vi "working-HostControl_Main.vi"() -> ()   [LabVIEW 2013]
uses:
  Messages.ctl
  PolarCoordTdef.ctl
  GainsTDef.ctl
  Support VIs/setpointCluster.ctl
  <vilib>/MakerHub/KinectOne/Private/Initialize Image [Color].vi
  <vilib>/MakerHub/PS4-Controller/Public/Open First Controller.vi
  Support VIs/bodyGlobal.vi
  <vilib>/MakerHub/KinectOne/KinectOne.lvlib
  <vilib>/MakerHub/PS4-Controller/LMH-PS4.lvlib
panel:
  in  "Reference Colour":u32(colorbox)
  in  "Argument Setpoint":dbl
  in  "Modulus Setpoint":dbl=1.8
  out "Tracked?":bool
  out "index":i32
  in  "Detect Mode":u16(ring) items=["Desperate", "ColourMatch"]
  in  "Cancel Button":bool
  out "Image":T1(plugin-control)
  in  "Kd-Argument":dbl
  in  "Kc-Argument":dbl
  in  "Kd-Modulus":dbl
  in  "Kc-Modulus":dbl
  out "Mod":dbl
  out "Arg":dbl
  in  "IT'S TIME TO":bool
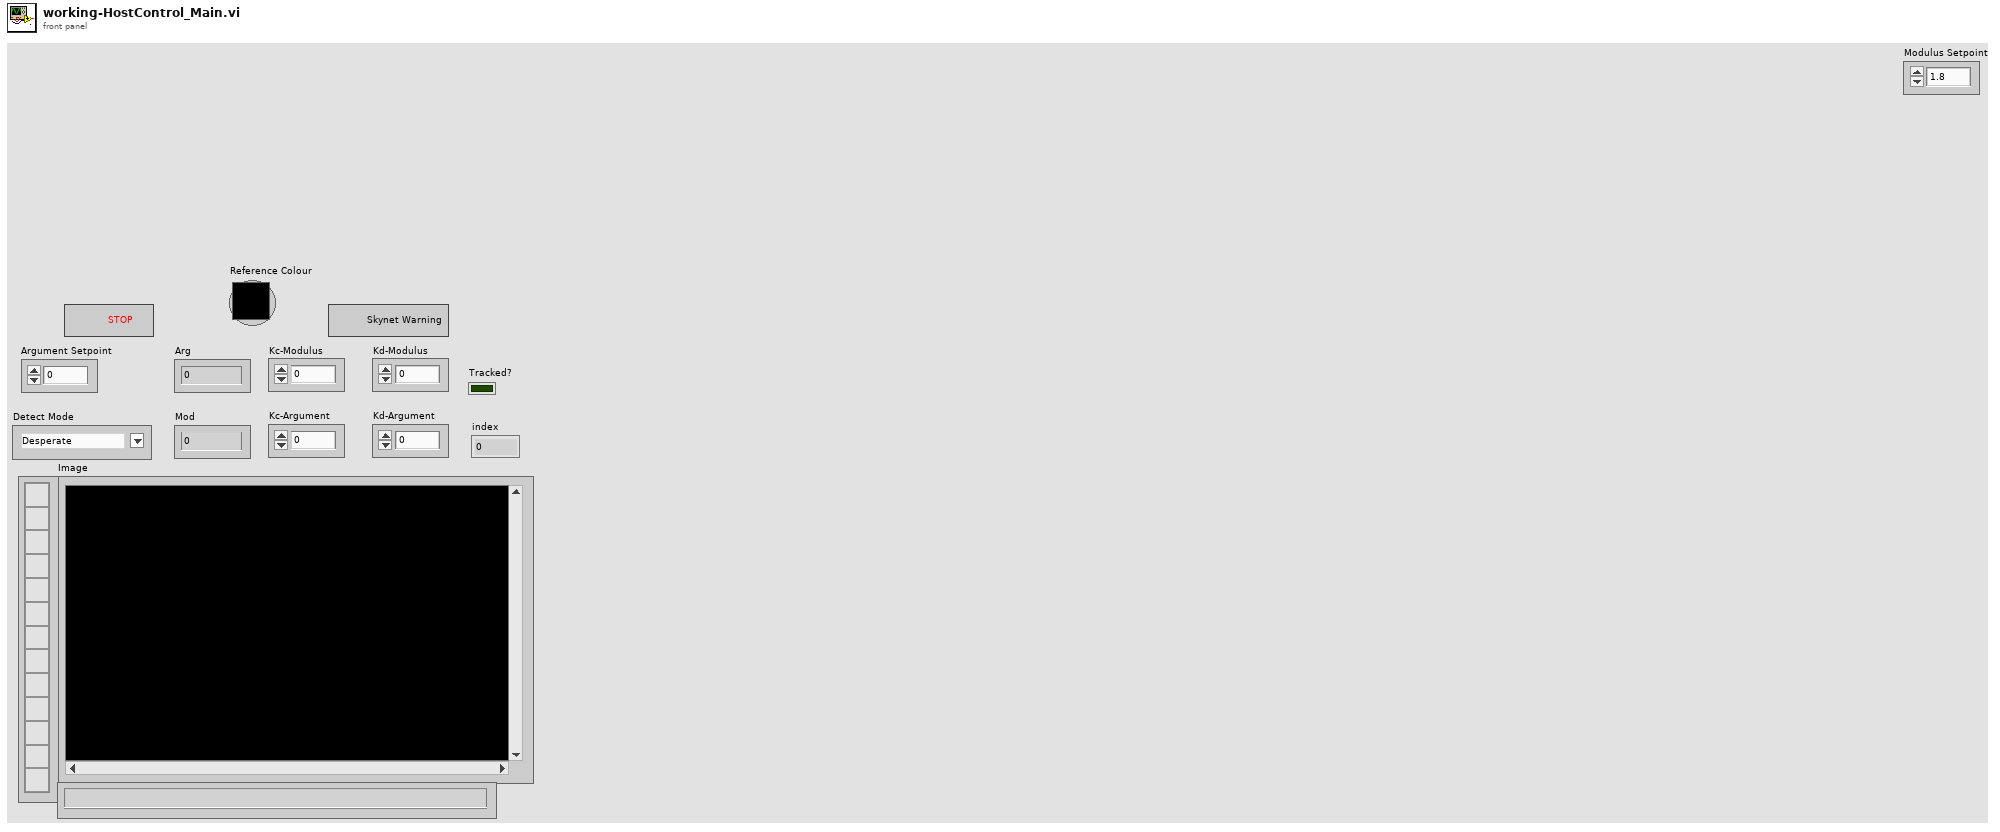
[diagram p1: front panel]
types:
  T1 = typedef "IMAQ Image.ctl" = refnum<image>
  T2 = typedef "Messages.ctl" = cluster{"message data":variant, "message type":enum16{"Stop", "PolarCoordinates", "Gains", "Setpoints"}}
  T3 = typedef "KinectOne.lvlib/KinectSensor References.ctl" = cluster{"KinectSensor":refnum<k24>, "MultiSourceFrameReader":refnum<k24>, "BodyFrameDataInterface":refnum<k24>}
  T4 = typedef "LMH-PS4.lvlib/PS4 Controller Ref.ctl" = cluster{"Controller Ref":refnum<k1>, "PS4 Events Ref":refnum<event-registration>, "Worker Ref":refnum<vi>}
  T5 = enum16{"Stop", "PolarCoordinates", "Gains", "Setpoints"}
  T6 = typedef "PolarCoordTdef.ctl" = cluster{"Argument":dbl, "Modulus":dbl, "trackedState":bool}
  T7 = typedef "KinectOne.lvlib/Joint Position.ctl" = cluster{"Camera Space":cluster{"X":dbl, "Y":dbl, "Z":dbl}, "Color Space":cluster{"X":dbl, "Y":dbl}, "Depth Space":cluster{"X":dbl, "Y":dbl}, "Tracking State":enum16{"NotTracked", "Inferred", "Tracked"}}
  T8 = typedef "setpointCluster.ctl" = cluster{"Modulus Setpoint":dbl, "Argument Setpoint":dbl}
  T9 = typedef "KinectOne.lvlib/BodyData.ctl" = cluster{"ClippedEdges":T10, "HandLeftConfidence":T11, "HandLeftState":T12, "HandRightConfidence":T13, "HandRightState":T14, "IsRestricted":bool, "IsTracked":bool, "JointOrientations":refnum<k24>, "Joints":refnum<k24>, "Lean":refnum<k24>, "LeanTrackingState":T15, "TrackingId":u64}
  T10 = typedef "KinectOne.lvlib/ClippedEdges.ctl" = enum16{"None", "Right", "Left", "Top", "Bottom"}
  T11 = typedef "KinectOne.lvlib/HandLeftConfidence.ctl" = enum16{"Low", "High"}
  T12 = typedef "KinectOne.lvlib/HandLeftState.ctl" = enum16{"Unknown", "NotTracked", "Open", "Closed", "Lasso"}
  T13 = typedef "KinectOne.lvlib/HandRightConfidence.ctl" = enum16{"Low", "High"}
  T14 = typedef "KinectOne.lvlib/HandRightState.ctl" = enum16{"Unknown", "NotTracked", "Open", "Closed", "Lasso"}
  T15 = typedef "KinectOne.lvlib/LeanTrackingState.ctl" = enum16{"NotTracked", "Inferred", "Tracked"}
  T16 = typedef "GainsTDef.ctl" = cluster{"Kc-Modulus":dbl, "Kd-Modulus":dbl, "Kc-Argument":dbl, "Kd-Argument":dbl}
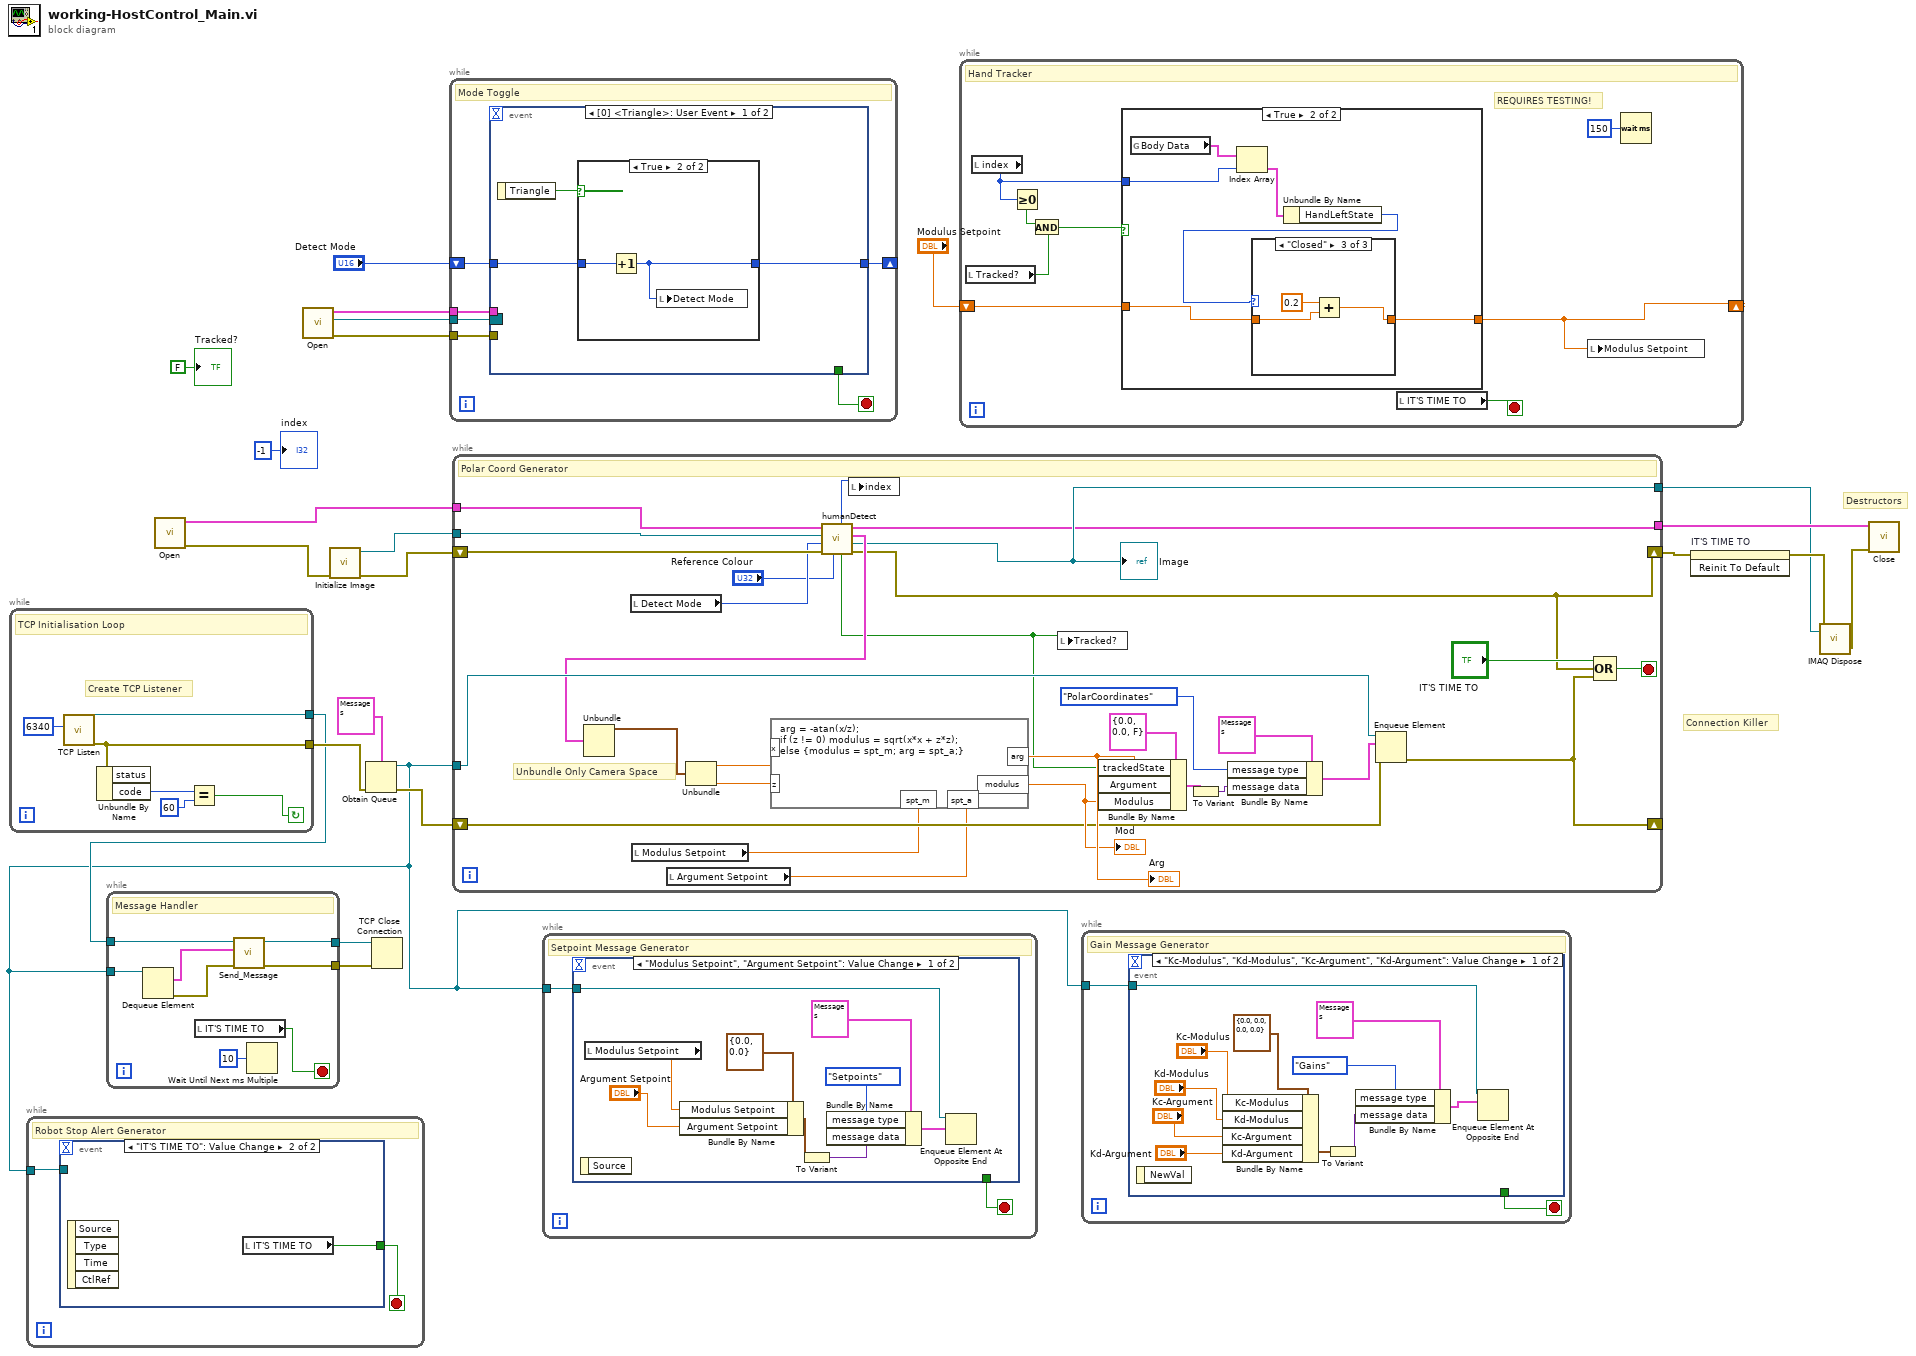
[diagram p0: block diagram]
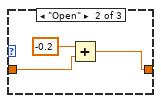
[diagram p4: hidden frame]
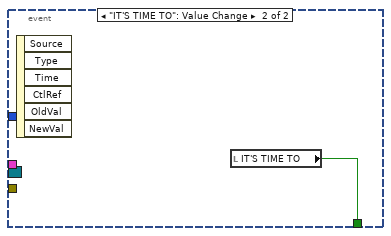
[diagram p6: hidden frame]
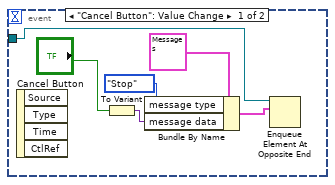
[diagram p7: hidden frame]
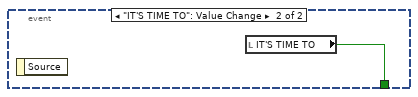
[diagram p8: hidden frame]
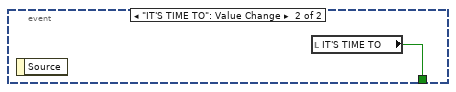
[diagram p9: hidden frame]
diagram:
  # "Connection Killer"
  # "Destructors"
  n1 = while {
    tunnel: [w28] -> w15
    tunnel: [w27] -> w18
    stop <- w24 continue-if-true
    # "Create TCP Listener"
    # "TCP Initialisation Loop"
    n2 = call <vilib>:"TCP Listen.vi"("port"=u16 6340) -> ("error out"=w27:errorcluster, "connection ID"=w28:refnum<k5>)  [unwired: 6 in, 3 out]
    n3 = Unbundle By Name(w27) -> ("code"=w26:i32)  [unwired: 1 out]
    n4 = Equal?(x=w26, y=60) -> (x = y?=w24:bool)
  }
  n5 = call <vilib>:"Open.vi"() -> ("Error Out"=w23:errorcluster, "KinectSensor References out"=w4:T3)  [unwired: 10 in]
  n6 = call-poly <vilib>:"Open.vi"() -> ("Error Out"=w6:errorcluster, "Event Registration Refnum"=w7:refnum<event-registration>, "PS4 Controller Ref"=w8:T4)  [unwired: 9 in]
  n7 = call-poly <vilib>:"Initialize Image.vi"("Error In"=w23) -> ("Error Out"=w22:errorcluster, "Color Image"=w21:T1)  [unwired: 9 in]
  n8 = Obtain Queue(element data type=T2 {"message data"=variant, "message type"=enum."Stop"} ("message"), error in (no error)=w18) -> (queue out=w12:refnum<queue>, error out=w17:errorcluster)  [unwired: 3 in, 1 out]
  n9 = while {
    tunnel: w12 -> [w31]
    stop <- w30 stop-if-true
    # "Robot Stop Alert Generator"
    n10 = event shown="[1] \"IT'S TIME TO\": Value Change" {
      selector: _ -> [_ _]
      dyn-events: _ -> [_ _]
      timeout: _ -> [_ _]
      tunnel: w31 -> [w35 _]
      tunnel: [_ w38] -> w30
      event "Cancel Button": Value Change {
        n11 = event-data() -> ()  [unwired: 1 in, 4 out]
        n12 = To Variant(anything="Cancel Button") -> (Variant=w34:variant)
        n13 = Bundle By Name(cluster=T2 {"message data"=variant, "message type"=enum."Stop"} ("message"), "message type"=T5."Stop", "message data"=w34) -> (w33:T2)
        n14 = Enqueue Element At Opposite End(queue=w35, element=w33) -> ()  [unwired: 2 in, 3 out]
      }
      event "IT'S TIME TO": Value Change {
        n15 = event-data() -> ()  [unwired: 1 in, 4 out]
        n16 = local read "IT'S TIME TO"() -> (w38:bool)
      }
    }
  }
  n17 = while {
    tunnel: w15 -> [w46]
    tunnel: w12 -> [w45]
    tunnel: [w41] -> w14
    tunnel: [w40] -> w13
    stop <- w39 stop-if-true
    # "Message Handler"
    n18 = Dequeue Element(queue=w45) -> (element=w44:T2, error out=w43:errorcluster)  [unwired: 2 in, 2 out]
    n19 = local read "IT'S TIME TO"() -> (w39:bool)
    n20 = call "Send_Message.vi"("error in (no error)"=w43, "message"=w44, "connection ID"=w46) -> ("error out (no error)"=w40:errorcluster, "connection ID 2"=w41:refnum<k5>)  [unwired: 7 in]
    n21 = Wait Until Next ms Multiple(millisecond multiple=u32 10 ("milliseconds to wait")) -> ()  [unwired: 1 out]
  }
  n22 = TCP Close Connection(connection ID=w14, error in (no error)=w13) -> ()  [unwired: 1 in, 2 out]
  n23 = while {
    tunnel: w8 -> [w52]
    tunnel: w7 -> [w50]
    tunnel: w6 -> [w51]
    shift-right: [w48] -> _
    shift-left: "Detect Mode" -> [w49]
    stop <- w47 stop-if-true
    # "Mode Toggle"
    n24 = event shown="[0] <Triangle>: User Event" {
      selector: w50 -> [_ _]
      dyn-events: _ -> [_ _]
      timeout: _ -> [_ _]
      tunnel: w52 -> [_ _]
      tunnel: w51 -> [_ _]
      tunnel: w49 -> [w54 _]
      tunnel: [w53 _] -> w48
      tunnel: [_ w59] -> w47
      event User Event {
        n25 = event-data() -> ("Triangle"=w55:bool)  [unwired: 1 in]
        n26 = case shown="True" w55 {
          tunnel: w54 -> [w56 w58]
          tunnel: [w56 w57] -> w53
          frame False {
          }
          frame True {
            n27 = Increment(x=w58) -> (x+1=w57:u16)
            n28 = local write "Detect Mode"(w57) -> ()
          }
        }
      }
      event "IT'S TIME TO": Value Change {
        n29 = event-data() -> ()  [unwired: 1 in, 6 out]
        n30 = local read "IT'S TIME TO"() -> (w59:bool)
      }
    }
  }
  n31 = while {
    tunnel: w4 -> [w72]
    tunnel: w21 -> [w71]
    shift-right: [w69] -> w11
    shift-left: w22 -> [w68]
    tunnel: [w64] -> w20
    shift-right: [w74] -> _
    shift-left: w17 -> [w75]
    tunnel: w12 -> [w73]
    tunnel: [w67] -> w9
    stop <- w81 stop-if-true
    # "Unbundle Only Camera Space"
    # "Polar Coord Generator"
    n32 = local read "Detect Mode"() -> (w65:u16)
    n33 = local read "Modulus Setpoint"() -> (w66:dbl)
    n34 = local read "Argument Setpoint"() -> (w61:dbl)
    n35 = call "humanDetect.vi"("Reference Colour"="Reference Colour", "Error In"=w68, "Enum"=w65, "Tracker"=w71, "KinectSensor References in"=w72) -> ("Error Out"=w69:errorcluster, "Image"=w67:T1, "Joint Position"=w70:T7, "KinectSensor References"=w64:T3, "istracked"=w62:bool, "index"=w63:i32)  [unwired: 1 in]
    "Image" <- w67
    n36 = Unbundle(w70) -> ("Camera Space"=w88:cluster{"X":dbl, "Y":dbl, "Z":dbl})  [unwired: 3 out]
    n37 = Unbundle(w88) -> ("X"=w83:dbl, "Z"=w82:dbl)  [unwired: 1 out]
    n38 = formula code="arg = -atan(x/z);\nif (z != 0) modulus = sqrt(x*x + z*z);\nelse {modulus = spt_m; arg = spt_a;}"("x"=w83, "z"=w82, "spt_m"=w66, "spt_a"=w61) -> ("arg"=w80:dbl, "modulus"=w79:dbl)
    "Arg" <- w80
    "Mod" <- w79
    n39 = local write "index"(w63) -> ()
    n40 = local write "Tracked?"(w62) -> ()
    n41 = Bundle By Name(cluster=T6 {"Argument"=0.0, "Modulus"=0.0, "trackedState"=FALSE}, "trackedState"=w62, "Argument"=w80, "Modulus"=w79) -> (w84:T6)
    n42 = To Variant(anything=w84) -> (Variant=w85:variant)
    n43 = Bundle By Name(cluster=T2 {"message data"=variant, "message type"=enum."Stop"} ("message"), "message type"=T5."PolarCoordinates", "message data"=w85) -> (w76:T2)
    n44 = Enqueue Element(queue=w73, element=w76, error in (no error)=w75) -> (error out=w74:errorcluster)  [unwired: 1 in, 2 out]
    n45 = Compound Arithmetic op=OR("IT'S TIME TO", w69, w74) -> (w81:bool)
  }
  n46 = while {
    tunnel: w12 -> [w90]
    stop <- w89 stop-if-true
    # "Setpoint Message Generator"
    n47 = event shown="[0] \"Modulus Setpoint\", \"Argument Setpoint\": Value Change" {
      selector: _ -> [_ _]
      dyn-events: _ -> [_ _]
      timeout: _ -> [_ _]
      tunnel: w90 -> [w94 _]
      tunnel: [_ w100] -> w89
      event "Modulus Setpoint", "Argument Setpoint": Value Change {
        n48 = event-data() -> ()  [unwired: 1 in, 1 out]
        n49 = local read "Modulus Setpoint"() -> (w92:dbl)
        n50 = Bundle By Name(cluster=T8 {"Modulus Setpoint"=0.0, "Argument Setpoint"=0.0} ("Setpoint Cluster"), "Modulus Setpoint"=w92, "Argument Setpoint"="Argument Setpoint") -> (w93:T8)
        n51 = To Variant(anything=w93) -> (Variant=w96:variant)
        n52 = Bundle By Name(cluster=T2 {"message data"=variant, "message type"=enum."Stop"} ("message"), "message type"=T5."Setpoints", "message data"=w96) -> (w95:T2)
        n53 = Enqueue Element At Opposite End(queue=w94, element=w95) -> ()  [unwired: 2 in, 3 out]
      }
      event "IT'S TIME TO": Value Change {
        n54 = event-data() -> ()  [unwired: 1 in, 1 out]
        n55 = local read "IT'S TIME TO"() -> (w100:bool)
      }
    }
  }
  n56 = while {
    shift-right: [w102] -> _
    shift-left: "Modulus Setpoint" -> [w103]
    stop <- w105 stop-if-true
    # "REQUIRES TESTING!"
    # "Hand Tracker"
    n57 = local read "Tracked?"() -> (w106:bool)
    n58 = local read "index"() -> (w104:i32)
    n59 = Greater Or Equal To 0?(x=w104) -> (x >= 0?=w107:bool)
    n60 = And(x=w107, y=w106) -> (x .and. y?=w108:bool)
    n61 = case shown="True" w108 {
      tunnel: w104 -> [_ w114]
      tunnel: w103 -> [w109 w111]
      tunnel: [w109 w110] -> w102
      frame False {
      }
      frame True {
        n62 = global read "bodyGlobal.vi" "Body Data"() -> (w115:T9[])
        n63 = Index Array(array=w115, index=w114) -> (element=w113:T9)
        n64 = Unbundle By Name(w113) -> ("HandLeftState"=w112:T12)
        n65 = case shown="\"Closed\"" w112 {
          tunnel: w111 -> [w116 w118 w121]
          tunnel: [w116 w117 w120] -> w110
          frame "Unknown", Default {
          }
          frame "Open" {
            n66 = Add(x=-0.2, y=w118) -> (x+y=w117:dbl)
          }
          frame "Closed" {
            n67 = Add(x=0.2, y=w121) -> (x+y=w120:dbl)
          }
        }
      }
    }
    n68 = local read "IT'S TIME TO"() -> (w105:bool)
    n69 = local write "Modulus Setpoint"(w102) -> ()
    n70 = Wait (ms)(milliseconds to wait=u32 150) -> ()  [unwired: 1 out]
  }
  n71 = while {
    tunnel: w12 -> [w124]
    stop <- w123 stop-if-true
    # "Gain Message Generator"
    n72 = event shown="[0] \"Kc-Modulus\", \"Kd-Modulus\", \"Kc-Argument\", \"Kd-Argument\": Value Change" {
      selector: _ -> [_ _]
      dyn-events: _ -> [_ _]
      timeout: _ -> [_ _]
      tunnel: w124 -> [w125 _]
      tunnel: [_ w136] -> w123
      event "Kc-Modulus", "Kd-Modulus", "Kc-Argument", "Kd-Argument": Value Change {
        n73 = event-data() -> ()  [unwired: 1 in, 1 out]
        n74 = Bundle By Name(cluster=T16 {"Kc-Modulus"=0.0, "Kd-Modulus"=0.0, "Kc-Argument"=0.0, "Kd-Argument"=0.0}, "Kc-Modulus"="Kc-Modulus", "Kd-Modulus"="Kd-Modulus", "Kc-Argument"="Kc-Argument", "Kd-Argument"="Kd-Argument") -> (w130:T16)
        n75 = To Variant(anything=w130) -> (Variant=w129:variant)
        n76 = Bundle By Name(cluster=T2 {"message data"=variant, "message type"=enum."Stop"} ("message"), "message type"=T5."Gains", "message data"=w129) -> (w126:T2)
        n77 = Enqueue Element At Opposite End(queue=w125, element=w126) -> ()  [unwired: 2 in, 3 out]
      }
      event "IT'S TIME TO": Value Change {
        n78 = event-data() -> ()  [unwired: 1 in, 1 out]
        n79 = local read "IT'S TIME TO"() -> (w136:bool)
      }
    }
  }
  n80 = invoke on="IT'S TIME TO" class="Bool (strict)" method="Reinit To Default"(error in=w11) -> (error out=w10:errorcluster)  [unwired: 2 in, 2 out]
  n81 = call "IMAQ Dispose"("Image"=w9, "error in (no error)"=w10) -> ("error out"=w19:errorcluster)  [unwired: 4 in]
  n82 = call <vilib>:"Close.vi"("Error In"=w19, "KinectSensor References"=w20) -> ()  [unwired: 9 in, 1 out]
  "index" <- -1 ("index")
  "Tracked?" <- FALSE ("Tracked?")
